vi "FTW-Endpoint-Multipart-Reply.vi"(0 "FTW Endpoint":refnum<class "FTW-Endpoint.lvclass">, 5 "Multipart Message":string[](array[string]), 7 "Timeout":i32 format="%dmsec", 11 "error in":errorcluster) -> (4 "FTW Endpoint out":refnum<class "FTW-Endpoint.lvclass">, 6 "Timed out?":bool, 15 "error out":errorcluster)   [LabVIEW 2012, in "FTW-Actor.lvlib" / "FTW-Endpoint.lvclass"]
uses:
  FTW-Endpoint.lvclass
panel:
  # "Inputs"
  # "Outputs"
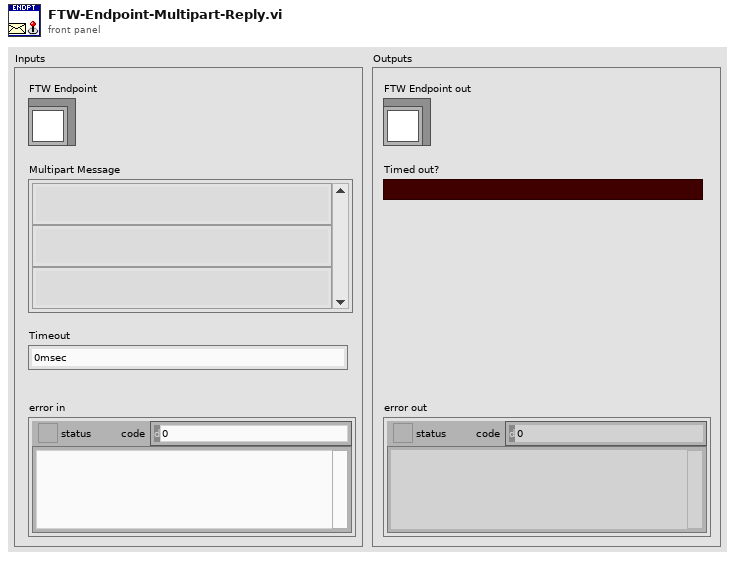
[diagram p1: front panel]
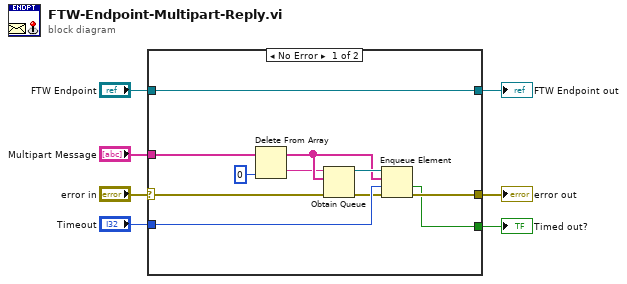
[diagram p0: block diagram]
diagram:
  n1 = case shown="No Error" "error in" {
    selector: "error in" -> [w14 w20]
    tunnel: [w18 w20] -> w7
    tunnel: [w15 w19] -> w5
    tunnel: "FTW Endpoint" -> [w15 w19]
    tunnel: "Multipart Message" -> [w11 _]
    tunnel: [w17 _] -> w2
    tunnel: "Timeout" -> [w16 _]
    frame No Error {
      n2 = Delete From Array(array=w11, index=0) -> (deleted portion=w8:string, array with subset deleted=w10:string[])  [unwired: 1 in]
      n3 = Obtain Queue(name (unnamed)=w8, element data type=w10, error in (no error)=w14) -> (queue out=w12:refnum<queue>, error out=w13:errorcluster)  [unwired: 2 in, 1 out]
      n4 = Enqueue Element(queue=w12, element=w10, timeout in ms (-1)=w16, error in (no error)=w13) -> (timed out?=w17:bool, error out=w18:errorcluster)  [unwired: 1 out]
    }
    frame Error {
    }
  }
  "error out" <- w7
  "FTW Endpoint out" <- w5
  "Timed out?" <- w2
